vi "Write DbMeasurement.lvclass.vi"(8 "error in (no error)":errorcluster, 10 "DbMeasurement.lvclass":refnum<class "DbMeasurement.lvclass">, 11 "BaseProducer in":refnum<class "BaseProducer.lvclass">) -> (0 "error out":errorcluster, 3 "BaseProducer out":refnum<class "BaseProducer.lvclass">)   [LabVIEW 2013, in "BaseProducer.lvclass"]
doc: "This accessor sets the DbMeasurement object in the producer object."
uses:
  BaseProducer.lvclass
  DbMeasurement/DbMeasurement.lvclass
  BaseProducer.lvclass/BaseProducer.ctl
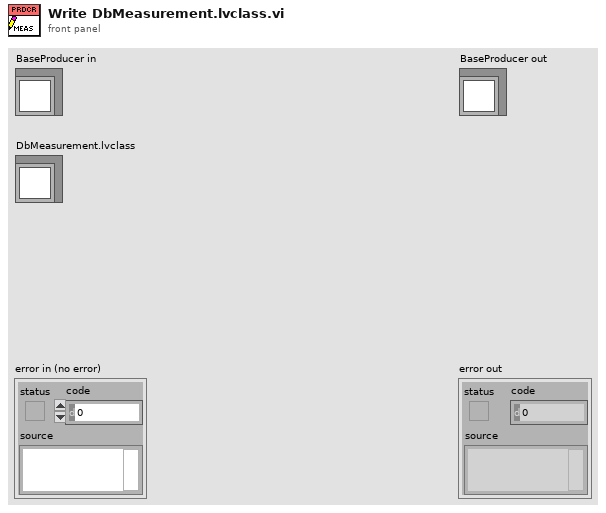
[diagram p1: front panel]
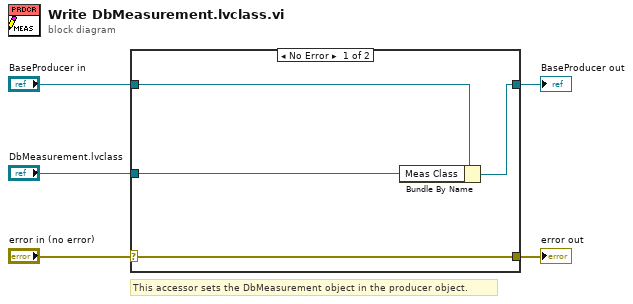
[diagram p0: block diagram]
diagram:
  # "This accessor sets the DbMeasurement object in the producer object."
  n1 = case shown="No Error" "error in (no error)" {
    selector: "error in (no error)" -> [w9 w10]
    tunnel: [w9 w10] -> w4
    tunnel: [w7 w11] -> w2
    tunnel: "BaseProducer in" -> [w8 w11]
    tunnel: "DbMeasurement.lvclass" -> [w6 _]
    frame No Error {
      n2 = Bundle By Name(cluster=w8, "Meas Class"=w6) -> (w7:refnum<class "BaseProducer.lvclass">)
    }
    frame Error {
    }
  }
  "error out" <- w4
  "BaseProducer out" <- w2
